vi "request.Read formatted request string.vi"(8 "error in (no error)":errorcluster, 11 "Request in":refnum<class "Request.lvclass">) -> (0 "error out":errorcluster, 2 "formatted request string":string, 3 "Request out":refnum<class "Request.lvclass">)   [LabVIEW 2016, in "Request.lvclass"]
uses:
  Request.lvclass
  <vilib>/NI/JSON Support for LabVIEW/JSON Data Classes/JSON Datatype/JSON Null.lvclass
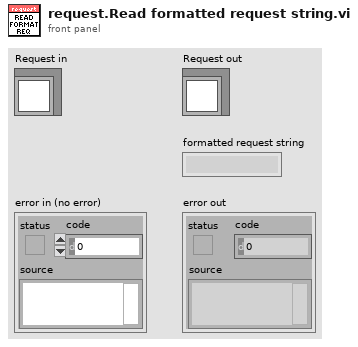
[diagram p1: front panel]
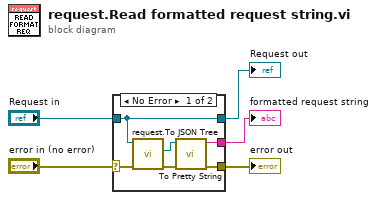
[diagram p0: block diagram]
diagram:
  n1 = case shown="No Error" "error in (no error)" {
    selector: "error in (no error)" -> [w6 w13]
    tunnel: [w7 w13] -> w4
    tunnel: [w11 w12] -> w2
    tunnel: "Request in" -> [w11 w12]
    tunnel: [w8 _] -> w1
    frame No Error {
      n2 = call "request.To JSON Tree.vi"("error in (no error)"=w6, "Request in"=w11) -> ("error out"=w10:errorcluster, "JSON out"=w9:refnum<class "JSON Null.lvclass">)  [unwired: 7 in, 1 out]
      n3 = call-dynamic "To Pretty String.vi"("error in (no error)"=w10, "JSON Datatype in"=w9) -> ("error out"=w7:errorcluster, "Pretty Print String"=w8:string)  [unwired: 8 in]
    }
    frame Error {
    }
  }
  "error out" <- w4
  "Request out" <- w2
  "formatted request string" <- w1
